vi "Gain and Probe Attenuation.vi"(0 "RedPitaya connection in":refnum<k5>, 2 "Probe Attenuation":dbl(ring) items=["0"=0.0, "0,01"=0.01, "0,02"=0.02, "0,05"=0.05, "0,1"=0.1, "0,2"=0.2, "0,5"=0.5, "1"=1.0, "2"=2.0, "5"=5.0, "10"=10.0, "20"=20.0, "50"=50.0, "100"=100.0, "200"=200.0, "500"=500.0, "1000"=1000.0], 3 "Input Gain":string(combo), 5 "error in":errorcluster, 8 "Channel #":u16(ring)=1 items=["Channel 1"=1, "Channel 2"=2], 12 "timeout ms (2000)":i32=2000) -> (14 "RedPitaya connection out":refnum<k5>, 19 "error out":errorcluster)   [LabVIEW 2010, in "RedPitaya.lvlib"]
doc: "Set Probe attenuation and Input gain."
uses:
  RedPitaya.lvlib
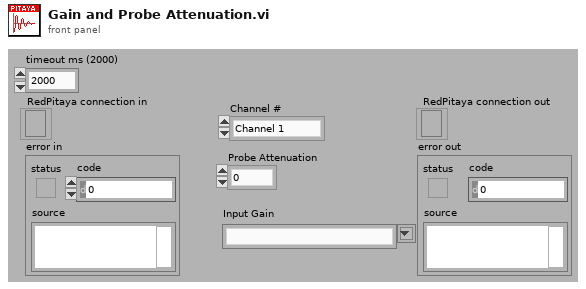
[diagram p1: front panel]
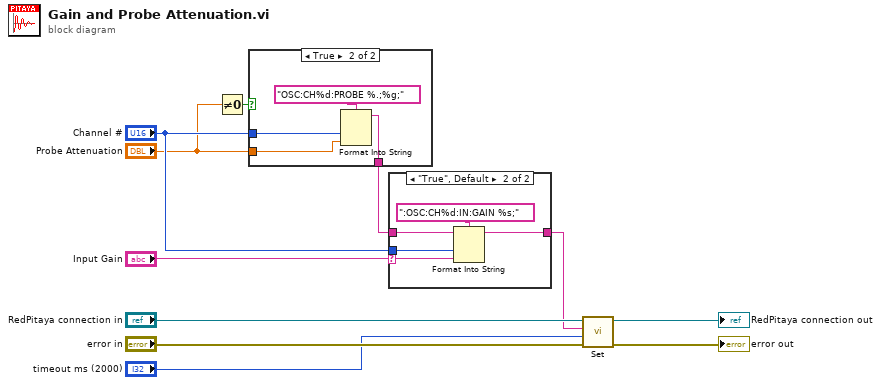
[diagram p0: block diagram]
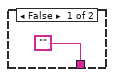
[diagram p3: hidden frame]
diagram:
  n1 = Not Equal To 0?(x="Probe Attenuation") -> (x != 0?=w4:bool)
  n2 = case shown="True" w4 {
    tunnel: "Probe Attenuation" -> [_ w15]
    tunnel: ["" w14] -> w7
    tunnel: "Channel #" -> [_ w13]
    frame False {
    }
    frame True {
      n3 = Format Into String(format string="OSC:CH%d:PROBE %.;%g;", w13, w15) -> (resulting string=w14:string)  [unwired: 2 in, 1 out]
    }
  }
  n4 = case shown="\"True\", Default" "Input Gain" {
    selector: "Input Gain" -> [_ w18]
    tunnel: w7 -> [w17 w22]
    tunnel: "Channel #" -> [_ w20]
    tunnel: [w17 w19] -> w5
    frame "" {
    }
    frame "True", Default {
      n5 = Format Into String(format string=":OSC:CH%d:IN:GAIN %s;", initial string=w22, w20, w18) -> (resulting string=w19:string)  [unwired: 1 in, 1 out]
    }
  }
  n6 = call "Set.vi"("error in"="error in", "timeout ms (2000)"="timeout ms (2000)", "SCPI Message"=w5, "RedPitaya connection in"="RedPitaya connection in") -> ("error out"=→"error out":errorcluster, "RedPitaya connection out"=→"RedPitaya connection out":refnum<k5>)  [unwired: 5 in, 1 out]
